vi "Read Type Name Path.vi"(8 "error in (no error)":errorcluster, 11 "_Template in":refnum<class "_Template.lvclass">) -> (0 "error out":errorcluster, 2 "Type Name Path":map{string, map{string, path}}(c390), 3 "_Template out":refnum<class "_Template.lvclass">)   [LabVIEW 2021, in "_Template.lvlib" / "_Template.lvclass"]
uses:
  _Template.lvclass
  _Template.lvclass/_Template.ctl
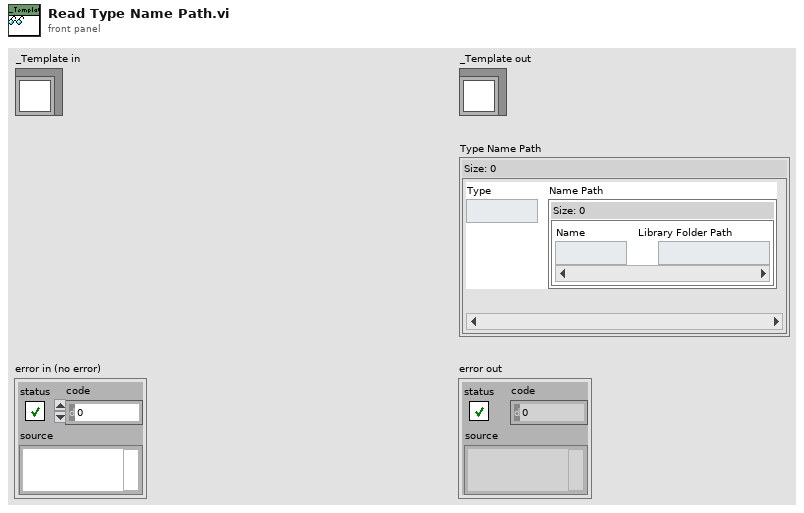
[diagram p1: front panel]
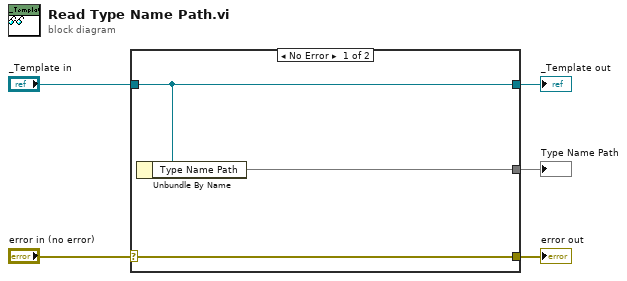
[diagram p0: block diagram]
diagram:
  n1 = case shown="No Error" "error in (no error)" {
    selector: "error in (no error)" -> [w8 w9]
    tunnel: [w8 w9] -> w4
    tunnel: [w7 w10] -> w2
    tunnel: "_Template in" -> [w7 w10]
    tunnel: [w6 _] -> w1
    frame No Error {
      n2 = Unbundle By Name(w7) -> ("Type Name Path"=w6:map{string, map{string, path}})
    }
    frame Error {
    }
  }
  "error out" <- w4
  "_Template out" <- w2
  "Type Name Path" <- w1
